vi "AI DAQ.vi"(11 "Queue ref":T1) -> ()   [LabVIEW 2022 SP3]
uses:
  Controls/All Queue.ctl
  Controls/DAQ case.ctl
  Controls/UI Data.ctl
  Controls/All Loop Status.ctl
  <vilib>/DAQmx/read.llb/DAQmx Read (Analog 1D Wfm NChan NSamp).vi
  Create Task/AI Create Task.vi
  <vilib>/DAQmx/configure/timing.llb/DAQmx Timing (Sample Clock).vi
  <vilib>/DAQmx/configure/trigger.llb/DAQmx Start Trigger (Time).vi
  Sub VI's/Global 1.vi
  <vilib>/DAQmx/miscellaneous.llb/DAQmx Fill In Error Info.vi
panel:
  # "TC channel list"
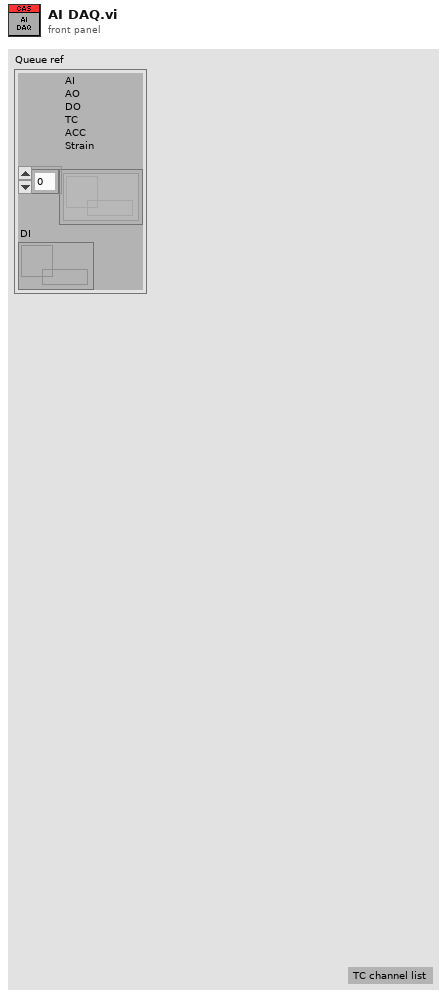
[diagram p1: front panel]
types:
  T1 = typedef "All Queue.ctl" = cluster{"AI\nAO\nDO\nTC\nACC\nStrain":refnum<queue>[], "DI":refnum<queue>}
  T2 = cluster{"in progress?":bool, "Queue ref":T1, "Start DAQ":refnum<notifier>, "UI Data":refnum<notifier>, "task out":refnum<k21>, "AI Ref":refnum<queue>, "SPC":i32}
  T3 = typedef "DAQ case.ctl" = enum16{"Initailise", "Create Task", "Polevent", "Acquire", "Stop DAQ", "Error", "Exit"}
  T4 = typedef "All Loop Status.ctl" = enum16{"AI", "AO", "DI", "DO", "TC", "Strain", "ACC", "RT", "Log"}
  T5 = enum16{"Init", "Read 'All'", "Read 'n'", "Read '1'", "Write '1'", "Write 'n'", "Write 'All'"}
  T6 = typedef "All Notifer.ctl" = cluster{"UI Data":refnum<notifier>, "Start DAQ":refnum<notifier>, "Start Log":refnum<notifier>}
  T7 = cluster{"Analog input":bool, "Analog Output":bool, "Digital input":bool, "Digital output":bool, "Thermocouple":bool, "Strain Gauge":bool, "Accelerometer":bool}
  T8 = typedef "Config.ctl" = cluster{"AO config":cluster{"Channel_Name":string, "Channel_Number":string, "Default_Value":dbl, "Units":string}[], "AI config":cluster{"Channel_Name":string, "Channel_Number":string, "Pre_Scale_min":dbl, "Pre_Scale_max":dbl, "Sensor_min":dbl, "Sensor_max":dbl, "Units":string}[], "DI config":cluster{"Channel_Name":string, "Channel_Number":string, "Default_Value":bool, "DI invert?":bool}[], "DO config":cluster{"Channel_Name":string, "Channel_Number":string, "Default_Value":bool, "DO invert?":bool}[], "TC config":cluster{"Channel_Name":string, "Channel_Number":string, "Pre_Scale_min":dbl, "Pre_Scale_max":dbl, "units":i32, " type":i32}[], "ACC config":cluster{"Channel_Name":string, "Channel_Number":string, "Pre_Scale_min":dbl, "Pre_Scale_max":dbl, "Terminal configuration":i32, "Sensitivity":dbl, "Sensitivity units":i32}[], "SG config":cluster{"Channel_Name":string, "Channel_Number":string, "Pre_Scale_min":dbl, "Pre_Scale_max":dbl}[], "Strain Gauge Settings":cluster{"poisson ratio":dbl, "nominal gage resistance":dbl, "gage factor":dbl}, "bridge information":cluster{"strain configuration":i32, "lead wire resistance":dbl, "initial bridge voltage":dbl, "voltage excitation source":i32, "voltage excitation value":dbl}, "Sample Rate":cluster{"AI Sample Rate":dbl, "AO Sample Rate":dbl, "DI Sample Rate":dbl, "TC Sample Rate":dbl, "DO Sample Rate":dbl, "SG Sample Rate":dbl, "ACC Sample Rate":dbl}}
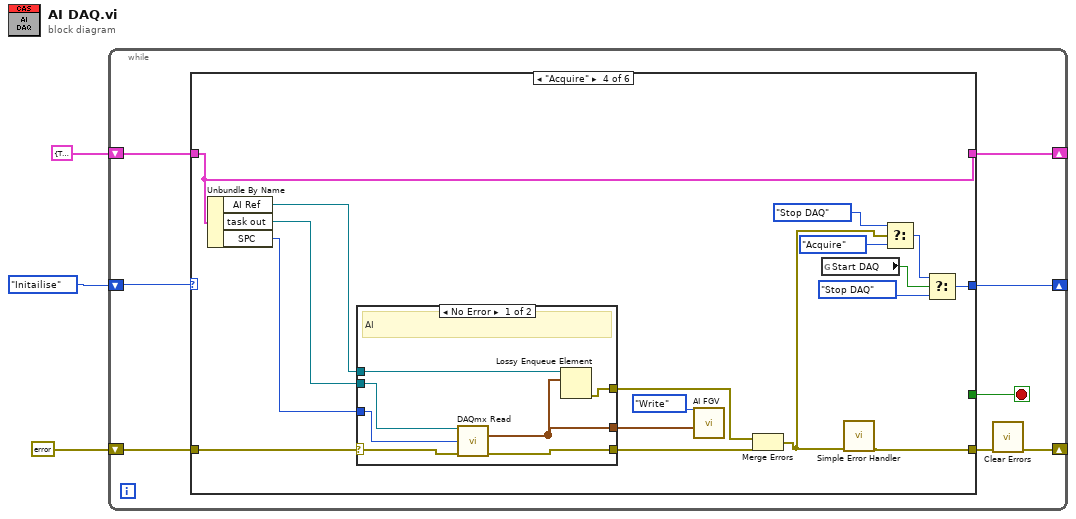
[diagram p0: block diagram]
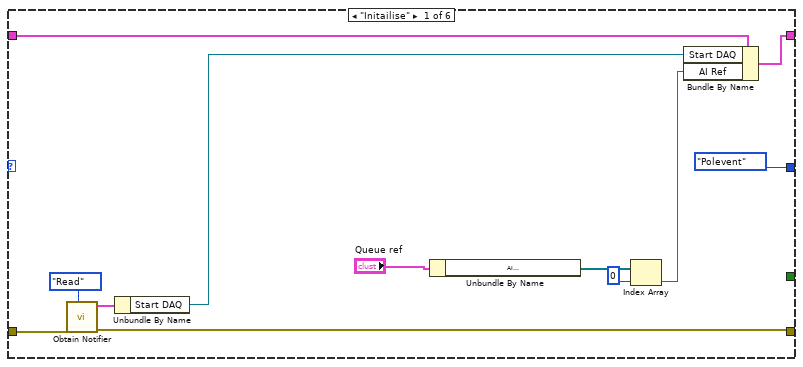
[diagram p2: hidden frame]
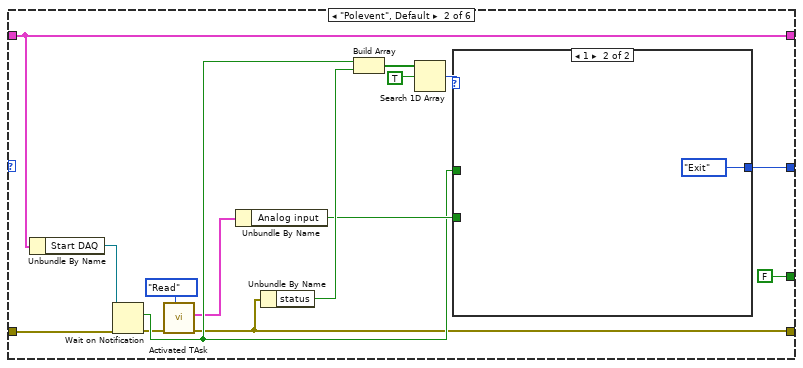
[diagram p3: hidden frame]
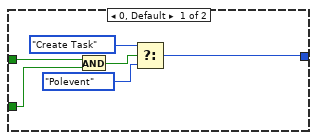
[diagram p4: hidden frame]
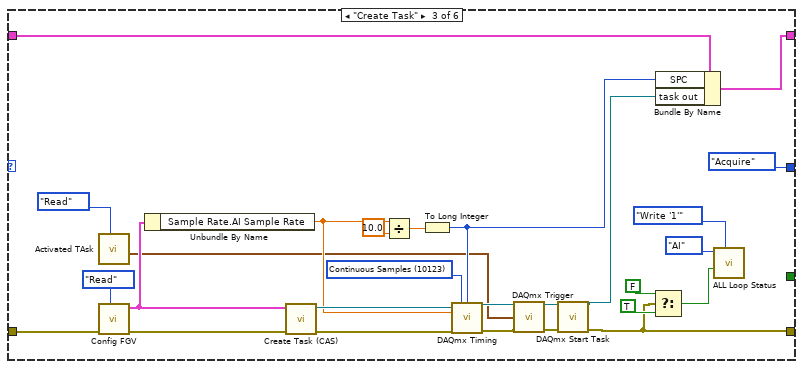
[diagram p5: hidden frame]
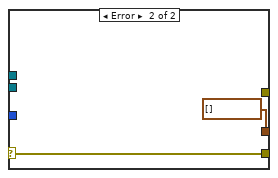
[diagram p6: hidden frame]
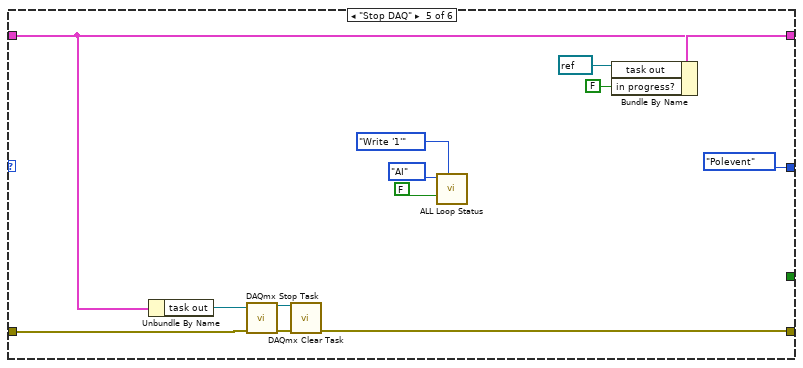
[diagram p7: hidden frame]
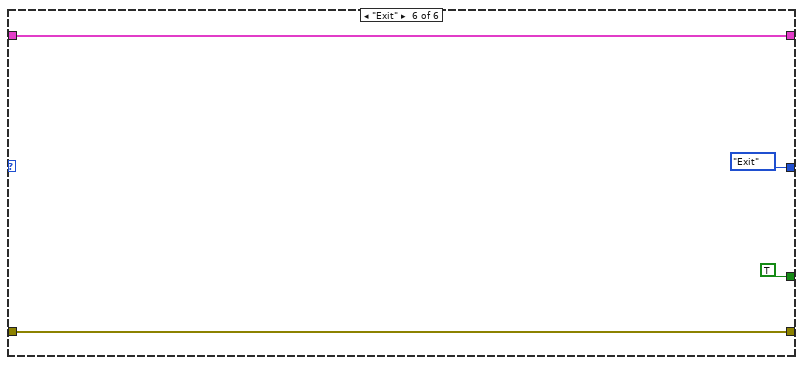
[diagram p8: hidden frame]
diagram:
  n1 = while {
    shift-right: [w4] -> _
    shift-left: errorcluster {"status"=FALSE, "code"=0, "source"=""} ("error out") -> [w10]
    shift-right: [w8] -> _
    shift-left: T2 {"in progress?"=TRUE, "Queue ref"={"AI\nAO\nDO\nTC\nACC\nStrain"=[], "DI"=refnum}, "Start DAQ"=refnum, "UI Data"=refnum, "task out"="", "AI Ref"=refnum, "SPC"=0} -> [w9]
    shift-right: [w7] -> _
    shift-left: DAQ_case."Initailise" -> [w6]
    stop <- w11 stop-if-true
    n2 = case shown="\"Acquire\"" w6 {
      tunnel: [_ FALSE _ _ _ TRUE] -> w11
      tunnel: w10 -> [w22 w27 w69 w82 w103 w115]
      tunnel: [w21 w25 w48 w77 w104 w115] -> w5
      tunnel: w9 -> [w19 w36 w71 w83 w108 w114]
      tunnel: [w17 w36 w70 w83 w109 w114] -> w8
      tunnel: [DAQ_case."Polevent" w37 DAQ_case."Acquire" w84 DAQ_case."Polevent" DAQ_case."Exit"] -> w7
      frame "Initailise" {
        n3 = call "Obtain Notifier.vi"("Case"=enum16{"Obtain", "Read"}."Read", "error in (no error)"=w22) -> ("error out"=w21:errorcluster, "notifiers out"=w20:T6)  [unwired: 8 in]
        n4 = Unbundle By Name(w20) -> ("Start DAQ"=w18:refnum<notifier>)
        n5 = Unbundle By Name("Queue ref") -> ("AI\nAO\nDO\nTC\nACC\nStrain"=w14:refnum<queue>[])
        n6 = Index Array(array=w14, index=0) -> (element=w13:refnum<queue>)
        n7 = Bundle By Name(cluster=w19, "Start DAQ"=w18, "AI Ref"=w13) -> (w17:T2)
      }
      frame "Polevent", Default {
        n8 = Unbundle By Name(w36) -> ("Start DAQ"=w35:refnum<notifier>)
        n9 = Wait on Notification(notifier=w35, error in (no error)=w27) -> (notification=w28:bool, error out=w26:errorcluster)  [unwired: 2 in, 2 out]
        n10 = call "Activated TAsk.vi"("Enum"=enum16{"Read", "Write"}."Read", "error in (no error)"=w26) -> ("error out"=w25:errorcluster, "Activate Task 2"=w24:T7)  [unwired: 7 in, 1 out]
        n11 = Unbundle By Name(w24) -> ("Analog input"=w29:bool)
        n12 = Unbundle By Name(w25) -> ("status"=w34:bool)
        n13 = Build Array(w28, w34) -> (w33:bool[])
        n14 = Search 1D Array(1D array=w33, element=TRUE) -> (index of element=w31:i32)  [unwired: 1 in]
        n15 = case shown="1" w31 {
          tunnel: [w43 DAQ_case."Exit"] -> w37
          tunnel: w29 -> [w40 _]
          tunnel: w28 -> [w39 _]
          frame 0, Default {
            n16 = And(x=w39, y=w40) -> (x .and. y?=w41:bool)
            n17 = Select(t=DAQ_case."Create Task", s=w41, f=DAQ_case."Polevent") -> (s? t:f=w43:T3)
          }
          frame 1 {
          }
        }
      }
      frame "Create Task" {
        w54 = 10123 items=["Finite Samples"=10178, "Continuous Samples"=10123, "Hardware Timed Single Point"=12522] ("sample mode")
        n18 = call "Activated TAsk.vi"("Enum"=enum16{"Read", "Write"}."Read") -> ("Start Time"=w49:timestamp)  [unwired: 8 in, 2 out]
        n19 = call "Config FGV.vi"("Enum"=enum16{"Read", "Write"}."Read", "error in (no error)"=w69) -> ("error out"=w66:errorcluster, "Data"=w58:T8)  [unwired: 8 in]
        n20 = Unbundle By Name(w58) -> ("Sample Rate.AI Sample Rate"=w55:dbl)
        n21 = call-poly "Create Task (CAS).vi"("error in"=w66, "Config"=w58) -> ("error out"=w64:errorcluster, "AI Task"=w65:refnum<k21>)  [unwired: 7 in, 1 out]
        n22 = Divide(x=w55, y=10.0) -> (x/y=w56:dbl)
        n23 = To Long Integer(number=w56) -> (32bit integer=w53:i32)
        n24 = call-poly <vilib>:"DAQmx Timing.vi"("task/channels in"=w65, "sample mode"=w54, "samples per channel"=w53, "rate"=w55, "error in"=w64) -> ("task out"=w50:refnum<k21>, "error out"=w52:errorcluster)  [unwired: 9 in]
        n25 = call-poly <vilib>:"DAQmx Trigger.vi"("task/channels in"=w50, "when"=w49, "error in"=w52) -> ("task out"=w47:refnum<k21>, "error out"=w51:errorcluster)  [unwired: 11 in]
        n26 = call <vilib>:"DAQmx Start Task.vi"("task/channels in"=w47, "error in"=w51) -> ("task out"=w46:refnum<k21>, "error out"=w48:errorcluster)  [unwired: 12 in]
        n27 = Select(t=FALSE, s=w48, f=TRUE) -> (s? t:f=w61:bool)
        n28 = Bundle By Name(cluster=w71, "SPC"=w53, "task out"=w46) -> (w70:T2)
        n29 = call "ALL Loop Status.vi"("Option"=T5."Write '1'", "Status"=w61, "Loop"=All_Loop_Status."AI") -> ()  [unwired: 6 in, 3 out]
      }
      frame "Acquire" {
        n30 = Unbundle By Name(w83) -> ("AI Ref"=w81:refnum<queue>, "task out"=w80:refnum<k21>, "SPC"=w76:i32)
        n31 = case shown="No Error" w82 {
          selector: w82 -> [w95 w98]
          tunnel: w80 -> [w94 _]
          tunnel: [w96 w98] -> w75
          tunnel: w81 -> [w92 _]
          tunnel: [w91 waveform(dbl)[] [] ("data")] -> w78
          tunnel: w76 -> [w93 _]
          tunnel: [w90 _] -> w73
          frame No Error {
            # "AI"
            n32 = call-poly <vilib>:"DAQmx Read.vi"("task/channels in"=w94, "number of samples per channel"=w93, "error in"=w95) -> ("data"=w91:waveform(dbl)[], "error out"=w96:errorcluster)  [unwired: 10 in, 1 out]
            n33 = Lossy Enqueue Element(queue=w92, element=w91) -> (error out=w90:errorcluster)  [unwired: 1 in, 3 out]
          }
          frame Error {
          }
        }
        n34 = call "AI FGV.vi"("AI data"=w78, "Enum"=enum16{"Read", "Write"}."Write") -> ()  [unwired: 9 in, 1 out]
        n35 = Merge Errors(w73, w75) -> (w74:errorcluster)
        n36 = global read "Global 1.vi" "Start DAQ"() -> (w87:bool)
        n37 = call <vilib>:"Simple Error Handler.vi"("error in (no error)"=w74) -> ("error out"=w77:errorcluster)  [unwired: 4 in, 4 out]
        n38 = Select(t=DAQ_case."Stop DAQ", s=w74, f=DAQ_case."Acquire") -> (s? t:f=w86:T3)
        n39 = Select(t=w86, s=w87, f=DAQ_case."Stop DAQ") -> (s? t:f=w84:T3)
      }
      frame "Stop DAQ" {
        n40 = Unbundle By Name(w108) -> ("task out"=w102:refnum<k21>)
        n41 = call <vilib>:"DAQmx Stop Task.vi"("task/channels in"=w102, "error in"=w103) -> ("task out"=w101:refnum<k21>, "error out"=w105:errorcluster)  [unwired: 12 in]
        n42 = call <vilib>:"DAQmx Clear Task.vi"("task in"=w101, "error in"=w105) -> ("error out"=w104:errorcluster)  [unwired: 13 in]
        n43 = call "ALL Loop Status.vi"("Option"=T5."Write '1'", "Status"=FALSE, "Loop"=All_Loop_Status."AI") -> ()  [unwired: 6 in, 3 out]
        n44 = Bundle By Name(cluster=w108, "task out"=refnum<k21> refnum, "in progress?"=FALSE) -> (w109:T2)
      }
      frame "Exit" {
      }
    }
    n45 = call <vilib>:"Clear Errors.vi"("error in (no error)"=w5) -> ("error out"=w4:errorcluster)  [unwired: 5 in, 1 out]
  }
